vi "Get Wire Info.vi"(11 "Wire":refnum<vi>) -> (2 "wire datatype":string, 3 "wire label":string)   [LabVIEW 2014]
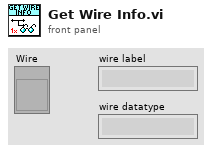
[diagram p1: front panel]
types:
  T1 = cluster{"wire labels":string[], "wire terminals datatypes":string[][]}
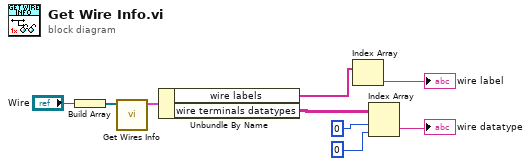
[diagram p0: block diagram]
diagram:
  n1 = Build Array("Wire") -> (w8:refnum<vi>[])
  n2 = call "Get Wires Info.vi"("connected\nwires refs."=w8) -> ("wires info cluster"=w7:T1)  [unwired: 10 in]
  n3 = Unbundle By Name(w7) -> ("wire labels"=w6:string[], "wire terminals datatypes"=w5:string[][])
  n4 = Index Array(array=w6) -> (element=→"wire label":string)  [unwired: 1 in]
  n5 = Index Array(array=w5, index (row)=0, index (col)=0 ("index (row)")) -> (element=→"wire datatype":string)
